vi "SGUI Set Single Integer By Label.vi"(6 "error in":errorcluster, 8 "label (empty)":string, 9 "format (empty)":string, 10 "value (none)":i32=-2147483648) -> (7 "error out":errorcluster, 11 "control reference out":refnum<vi>)   [LabVIEW 2020, in "varilib.lvlib"]
doc: "This VI sets value and format of numeric control designated by label name string. If empty format string is entered, format stays unchanged. If NaN value is entered, the value is not modified. \n\nThi VI ignores input errors (will execute anyway) however will generate error if any of the named controls is not found or writting to it fails (invalid type of control)."
uses:
  varilib.lvlib
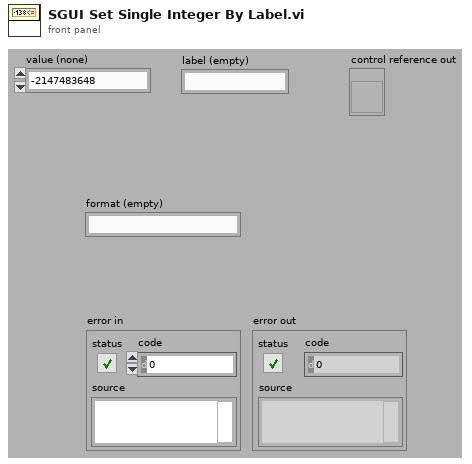
[diagram p1: front panel]
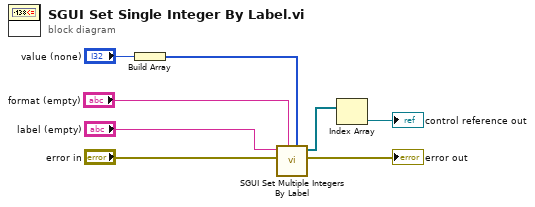
[diagram p0: block diagram]
diagram:
  n1 = Build Array("value (none)") -> (w1:i32[])
  n2 = call "SGUI Set Multiple Integers By Label.vi"("error in"="error in", "labels (empty)"="label (empty)", "format (empty)"="format (empty)", "integers (empty)"=w1) -> ("error out"=→"error out":errorcluster, "control references out"=w6:refnum<vi>[])  [unwired: 6 in]
  n3 = Index Array(array=w6) -> (element=→"control reference out":refnum<vi>)  [unwired: 1 in]
